vi "FGV_Tree Custom Symbols.vi"(7 "Operation":T1, 8 "error in (no error)":errorcluster, 9 "PicName":string, 10 "Files":path, 11 "tree refnum":refnum<vi>) -> (0 "error out":errorcluster, 2 "PicIndex":i32)   [LabVIEW 2017]
doc: "Loads graphics files from disk and assigns the images for use as custom symbols in the tree control."
uses:
  FV_Tree Custom Symbols.ctl
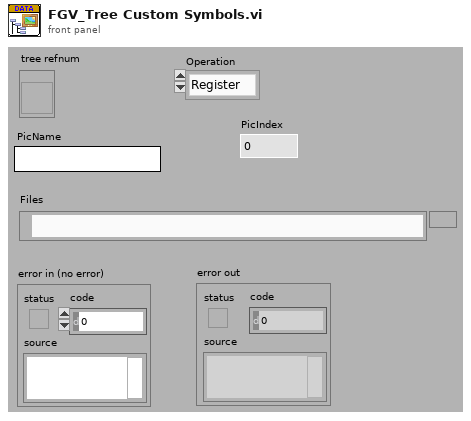
[diagram p1: front panel]
types:
  T1 = typedef "FV_Tree Custom Symbols.ctl" = enum16{"Register", "GetIndex"}
  T2 = typedef "imagedata.ctl" = cluster{"image type":i32, "image depth":i32, "image":u8[], "mask":u8[], "colors":u32[], "Rectangle":cluster{"left":i16, "top":i16, "right":i16, "bottom":i16}}
  T3 = cluster{string[], i32[], "All Files in Dir":path[], T2[]}
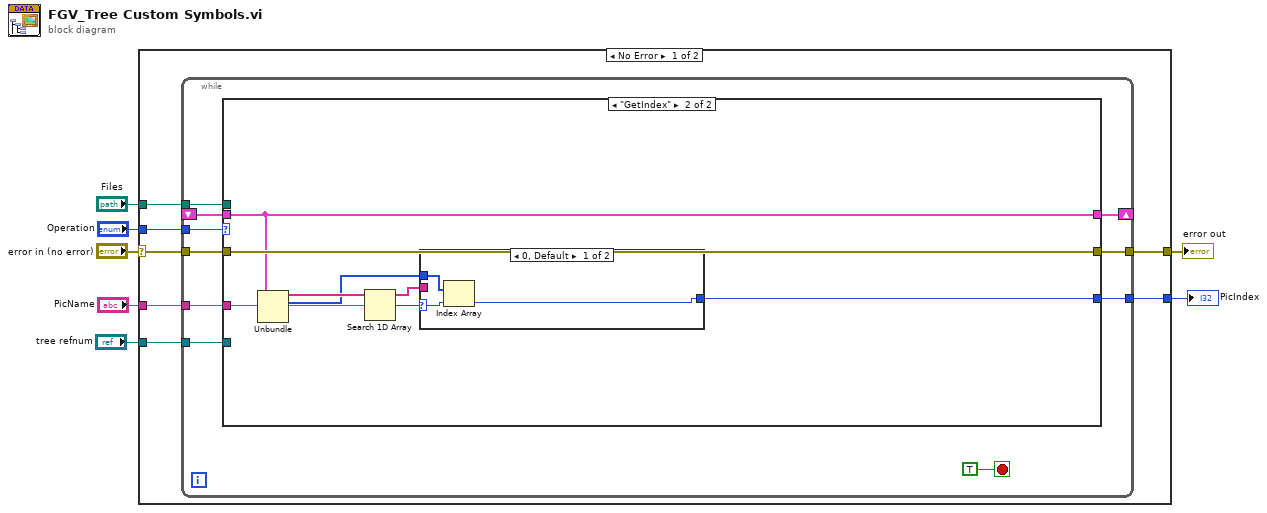
[diagram p0: block diagram]
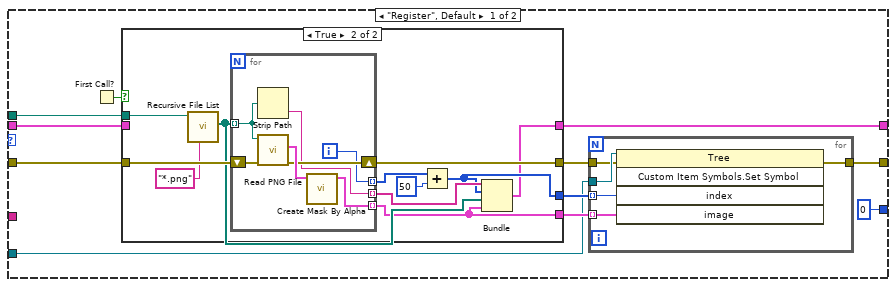
[diagram p2: hidden frame]
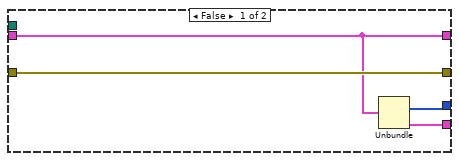
[diagram p3: hidden frame]
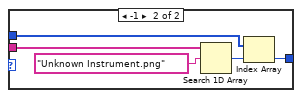
[diagram p4: hidden frame]
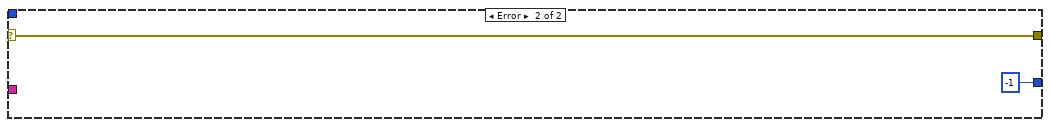
[diagram p5: hidden frame]
diagram:
  n1 = case shown="No Error" "error in (no error)" {
    selector: "error in (no error)" -> [w14 w79]
    tunnel: "tree refnum" -> [w12 _]
    tunnel: [w11 w79] -> w6
    tunnel: "Files" -> [w13 _]
    tunnel: "Operation" -> [w10 _]
    tunnel: "PicName" -> [w9 _]
    tunnel: [w8 -1] -> w1
    frame No Error {
      n2 = while {
        tunnel: w14 -> [w24]
        tunnel: w13 -> [w23]
        shift-right: [w21] -> _
        shift-left: _ -> [w20]
        tunnel: [w19] -> w11
        tunnel: w12 -> [w18]
        tunnel: w10 -> [w17]
        tunnel: w9 -> [w16]
        tunnel: [w15] -> w8
        stop <- TRUE stop-if-true
        n3 = case shown="\"GetIndex\"" w17 {
          tunnel: w24 -> [w35 w64]
          tunnel: w23 -> [w34 _]
          tunnel: [w32 w63] -> w21
          tunnel: w20 -> [w31 w63]
          tunnel: [w29 w64] -> w19
          tunnel: w18 -> [w26 _]
          tunnel: w16 -> [_ w66]
          tunnel: [0 w65] -> w15
          frame "Register", Default {
            n4 = First Call?() -> (First Call?: T/F=w33:bool)
            n5 = case shown="True" w33 {
              tunnel: [w44 w55] -> w30
              tunnel: w35 -> [w44 w54]
              tunnel: [w41 w47] -> w27
              tunnel: w34 -> [_ w53]
              tunnel: [w42 w49] -> w28
              tunnel: [w43 w45] -> w32
              tunnel: w31 -> [w43 _]
              frame False {
                n6 = Unbundle(w43) -> (w42:i32[], w41:T2[])  [unwired: 2 out]
              }
              frame True {
                n7 = call <vilib>:"Recursive File List.vi"("pattern"="*.png", "Folder Path"=w53) -> ("All Files in Dir"=w48:path[])  [unwired: 5 in, 4 out]
                n8 = for {
                  tunnel: w48 -> [w57] mode=indexing
                  tunnel: [w61] -> w47 mode=indexing
                  shift-right: [w59] -> w55
                  shift-left: w54 -> [w60]
                  tunnel: [w58] -> w52 mode=indexing
                  tunnel: [w56] -> w50 mode=indexing
                  i -> [w58]
                  n9 = Strip Path(path=w57) -> (name=w56:string)  [unwired: 1 out]
                  n10 = call <vilib>:"Read PNG File.vi"("error in (no error)"=w60, "path to PNG file"=w57) -> ("error out"=w59:errorcluster, "image data"=w62:T2)  [unwired: 7 in, 1 out]
                  n11 = call <vilib>:"Create Mask By Alpha.vi"("image data"=w62) -> ("masked image data"=w61:T2)  [unwired: 10 in]
                }
                n12 = Add(x=w52, y=50 ("索引")) -> (x+y=w49:i32[])
                n13 = Bundle(w50, w49, "All Files in Dir"=w48, w47) -> (w45:T3)  [unwired: 1 in]
              }
            }
            n14 = for {
              tunnel: w26 -> [w40]
              tunnel: w27 -> [w39] mode=indexing
              tunnel: w28 -> [w38] mode=indexing
              tunnel: w30 -> [w37]
              tunnel: [w36] -> w29
              n15 = invoke class="Tree" method="Custom Item Symbols.Set Symbol"(reference=w40, error in=w37, "index"=w38, "image"=w39) -> (error out=w36:errorcluster)  [unwired: 1 in, 4 out]
            }
          }
          frame "GetIndex" {
            n16 = Unbundle(w63) -> (w68:string[], w67:i32[])  [unwired: 2 out]
            n17 = Search 1D Array(1D array=w68, element=w66) -> (index of element=w69:i32)  [unwired: 1 in]
            n18 = case shown="0, Default" w69 {
              selector: w69 -> [w71 _]
              tunnel: w67 -> [w72 w74]
              tunnel: [w70 w73] -> w65
              tunnel: w68 -> [_ w77]
              frame 0, Default {
                n19 = Index Array(array=w72, index=w71) -> (element=w70:i32)
              }
              frame -1 {
                n20 = Search 1D Array(1D array=w77, element="Unknown Instrument.png" ("PicName")) -> (index of element=w75:i32)  [unwired: 1 in]
                n21 = Index Array(array=w74, index=w75) -> (element=w73:i32)
              }
            }
          }
        }
      }
    }
    frame Error {
    }
  }
  "error out" <- w6
  "PicIndex" <- w1
